vi "Mouli.vi"() -> ()   [LabVIEW 2020]
panel:
  in  "entrée d'erreur":errorcluster
  out "tableau":string[][](array[string])
  out "Tableau":string[][](array[string])
  in  "chemin":path
  # "RIGHT CLICK + EXPORT EXCEL"
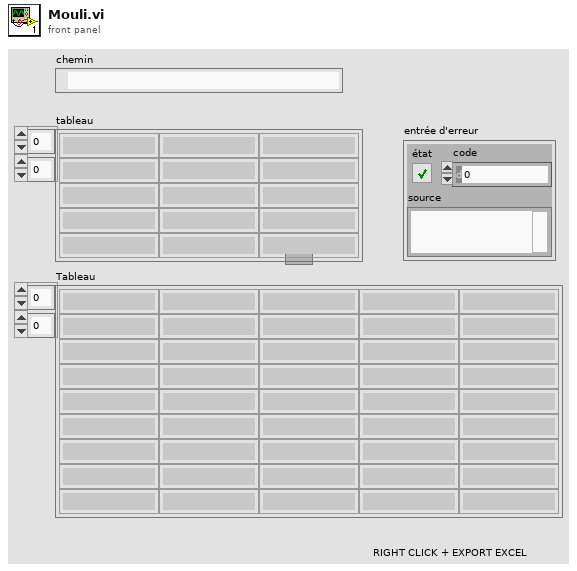
[diagram p1: front panel]
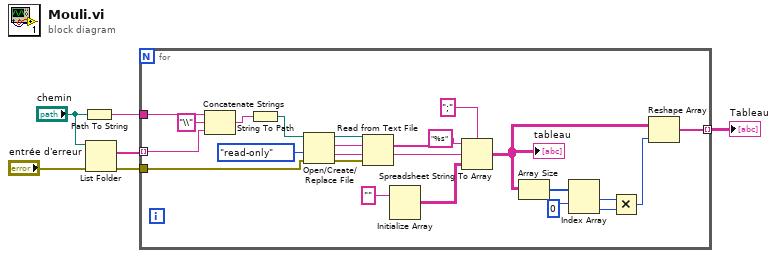
[diagram p0: block diagram]
diagram:
  n1 = Path To String(path="chemin") -> (string=w5:string)
  n2 = List Folder(path="chemin", error in="entrée d'erreur") -> (filenames=w4:string[], error out=w2:errorcluster)  [unwired: 2 in, 2 out]
  n3 = for {
    tunnel: w5 -> [w27]
    tunnel: w4 -> [w25] mode=indexing
    tunnel: [w13] -> w1 mode=indexing
    tunnel: w2 -> [w11]
    n4 = Concatenate Strings(w27, "\\" ("chaîne"), w25) -> (w24:string)
    n5 = String To Path(string=w24) -> (path=w23:path)
    n6 = Open/Create/Replace File(file path (use dialog)=w23, error in=w11, access (0:read/write)=enum16{"read/write", "read-only", "write-only"}."read-only" ("accès (0 : read/write)")) -> (refnum out=w22:refnum<file>, error out=w10:errorcluster)  [unwired: 3 in, 1 out]
    n7 = Read from Text File(file (use dialog)=w22, error in=w10) -> (text=w7:string)  [unwired: 2 in, 3 out]
    n8 = Initialize Array("") -> (w20:string[][])  [unwired: 2 in]
    n9 = Spreadsheet String To Array(delimiter (Tab)=";" ("séparateur (Tabulation)"), format string="%s" ("chaîne de format"), spreadsheet string=w7, array type (2D Dbl)=w20) -> (array=w15:string[][])
    "tableau" <- w15
    n10 = Array Size(array=w15) -> (size(s)=w17:i32[])
    n11 = Index Array(array=w17, index #1=0 ("indice")) -> (element #1=w9:i32, element #2=w16:i32)  [unwired: 1 in]
    n12 = Multiply(x=w9, y=w16) -> (x*y=w14:i32)
    n13 = Reshape Array(w15, w14) -> (w13:string[])
  }
  "Tableau" <- w1
